vi "Agilent VNA Read Identification.vi"(8 "error in (no error)":errorcluster, 11 "VISA Resource Name":refnum<visa-resource-name>) -> (0 "error out":errorcluster, 1 "Serial Number":string, 2 "Model Number":string, 3 "dup VISA Resource Name":refnum<visa-resource-name>, 5 "Firmware":string)   [LabVIEW 2011]
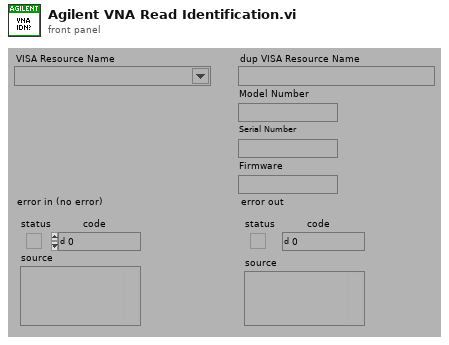
[diagram p1: front panel]
types:
  T1 = typedef "Agilent VNA Model.ctl" = enum16{"Not Supported", "8510X", "8719X", "8720X", "8722X", "8753X", "ENA", "PNA", "Field Fox"}
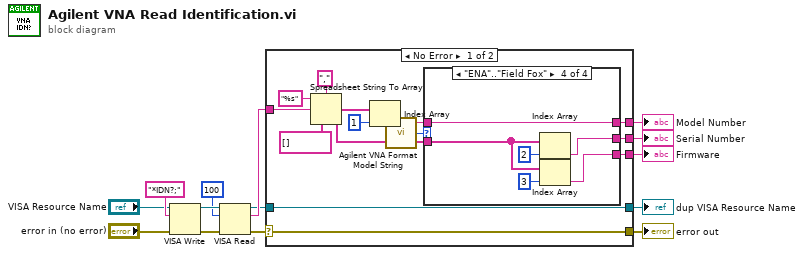
[diagram p0: block diagram]
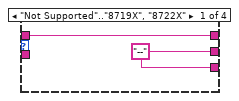
[diagram p2: hidden frame]
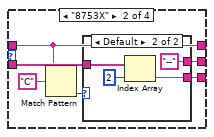
[diagram p3: hidden frame]
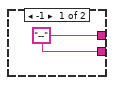
[diagram p4: hidden frame]
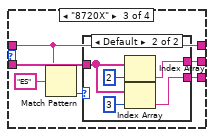
[diagram p5: hidden frame]
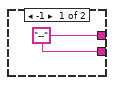
[diagram p6: hidden frame]
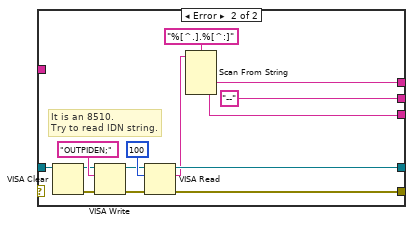
[diagram p7: hidden frame]
diagram:
  n1 = VISA Write(VISA resource name="VISA Resource Name", write buffer="*IDN?;", error in (no error)="error in (no error)") -> (VISA resource name out=w14:refnum<visa-resource-name>, error out=w12:errorcluster)  [unwired: 1 out]
  n2 = VISA Read(VISA resource name=w14, byte count=u32 100, error in (no error)=w12) -> (VISA resource name out=w5:refnum<visa-resource-name>, read buffer=w10:string, error out=w7:errorcluster)  [unwired: 1 out]
  n3 = case shown="No Error" w7 {
    selector: w7 -> [w26 _]
    tunnel: w10 -> [w20 _]
    tunnel: [w26 w67] -> w6
    tunnel: w5 -> [w27 w65]
    tunnel: [w27 w68] -> w4
    tunnel: [w19 w60] -> w3
    tunnel: [w18 "--"] -> w2
    tunnel: [w17 w59] -> w1
    frame No Error {
      n4 = Spreadsheet String To Array(delimiter (Tab)=",", format string="%s", spreadsheet string=w20, array type (2D Dbl)=string[] []) -> (array=w21:string[])
      n5 = Index Array(array=w21, index=1) -> (element=w15:string)
      n6 = call "Agilent VNA Format Model String.vi"("Model"=w15) -> ("Model"=w16:T1)
      n7 = case shown="\"ENA\"..\"Field Fox\"" w16 {
        tunnel: [w28 w30 w43 w53] -> w19
        tunnel: w21 -> [_ w31 w46 w56]
        tunnel: [w29 w33 w45 w55] -> w18
        tunnel: [w29 w32 w44 w54] -> w17
        tunnel: w15 -> [w28 w30 w43 w53]
        frame "Not Supported".."8719X", "8722X" {
          w29 = "--"
        }
        frame "8753X" {
          n8 = Match Pattern(string=w30, regular expression="C") -> (offset past match=w35:i32)  [unwired: 4 out]
          n9 = case shown="Default" w35 {
            tunnel: w31 -> [_ w39]
            tunnel: [w36 "--"] -> w33
            tunnel: [w36 w38] -> w32
            frame -1 {
              w36 = "--"
            }
            frame Default {
              n10 = Index Array(array=w39, index=2) -> (element=w38:string)
            }
          }
        }
        frame "8720X" {
          n11 = Match Pattern(string=w43, regular expression="ES") -> (offset past match=w42:i32)  [unwired: 4 out]
          n12 = case shown="Default" w42 {
            tunnel: w46 -> [_ w50]
            tunnel: [w47 w49] -> w45
            tunnel: [w47 w48] -> w44
            frame -1 {
              w47 = "--"
            }
            frame Default {
              n13 = Index Array(array=w50, index=2) -> (element=w49:string)
              n14 = Index Array(array=w50, index=3) -> (element=w48:string)
            }
          }
        }
        frame "ENA".."Field Fox" {
          n15 = Index Array(array=w56, index=2) -> (element=w55:string)
          n16 = Index Array(array=w56, index=3) -> (element=w54:string)
        }
      }
    }
    frame Error {
      # "It is an 8510.\nTry to read IDN string."
      n17 = VISA Clear(VISA resource name=w65) -> (VISA resource name out=w64:refnum<visa-resource-name>, error out=w63:errorcluster)  [unwired: 1 in]
      n18 = VISA Write(VISA resource name=w64, write buffer="OUTPIDEN;", error in (no error)=w63) -> (VISA resource name out=w69:refnum<visa-resource-name>, error out=w71:errorcluster)  [unwired: 1 out]
      n19 = VISA Read(VISA resource name=w69, byte count=u32 100, error in (no error)=w71) -> (VISA resource name out=w68:refnum<visa-resource-name>, read buffer=w61:string, error out=w67:errorcluster)  [unwired: 1 out]
      n20 = Scan From String(format string="%[^.].%[^:]", input string=w61) -> (output 1=w60:string, output 2=w59:string)  [unwired: 2 in, 5 out]
    }
  }
  "error out" <- w6
  "dup VISA Resource Name" <- w4
  "Model Number" <- w3
  "Serial Number" <- w2
  "Firmware" <- w1
